vi "_CSMObj-Obtain CSM.vi"(7 "Allowed Messages (Empty For All)":string[](array[string]), 8 "error in (no error)":errorcluster, 11 "Requested Name":string) -> (0 "error out":errorcluster, 3 "CSMQ Out":T1)   [LabVIEW 2017, in "Communicable State Machine.lvlib"]
uses:
  Communicable State Machine.lvlib
  _CSMObj.ctl
  _CSMObj-Info.ctl
  Typedef/_CSM_MODE.ctl
  _CSMObj-Refs.ctl
  _CSMObj-Data.ctl
  Typedef/_CSM_MSG_TYPE.ctl
  Priority Queue/Priority Queue.ctl
  Typedef/_Cross CSM State Data.ctl
  Typedef/_Cross CSM State Response.ctl
  Typedef/_CSM_Response Source Message.ctl
  Priority Queue/def-Data(LowPRI-Q).ctl
  _CSMObj-ModeData.ctl
  Typedef/_CSM Status Change Event Data.ctl
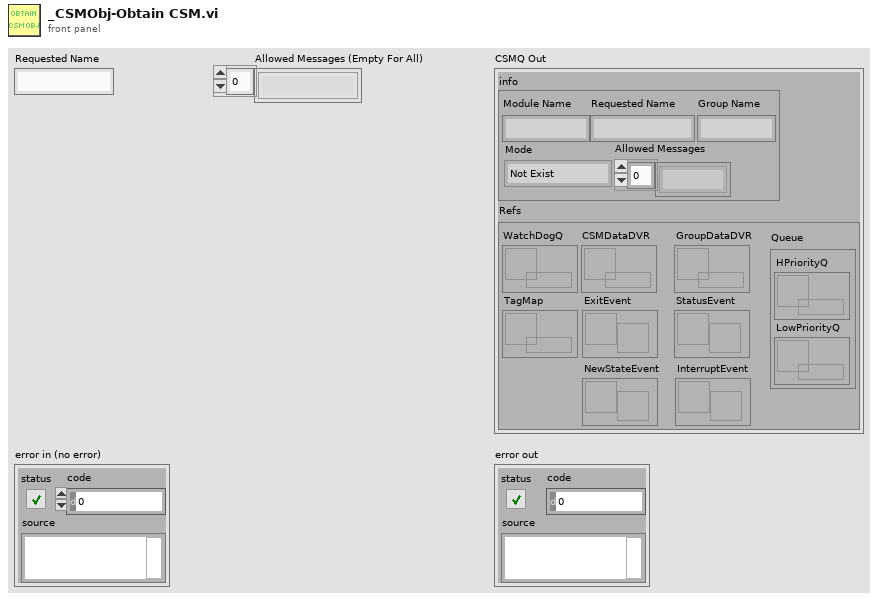
[diagram p1: front panel]
types:
  T1 = typedef "Communicable State Machine.lvlib/_CSMObj.ctl" = cluster{"info":T2, "Refs":T4}
  T2 = typedef "Communicable State Machine.lvlib/_CSMObj-Info.ctl" = cluster{"Module Name":string, "Requested Name":string, "Group Name":string, "Mode":T3, "Allowed Messages":string[]}
  T3 = typedef "Communicable State Machine.lvlib/_CSM_MODE.ctl" = enum16{"Not Exist", "Stand Alone", "CSM", "Worker", "Worker Agent", "Chain Node", "Chain"}
  T4 = typedef "Communicable State Machine.lvlib/_CSMObj-Refs.ctl" = cluster{"WatchDogQ":refnum<queue>, "CSMDataDVR":refnum<data-value>, "Queue":T5, "GroupDataDVR":refnum<data-value>, "TagMap":refnum<data-value>, "ExitEvent":refnum<user-event>, "NewStateEvent":refnum<user-event>, "StatusEvent":refnum<user-event>, "InterruptEvent":refnum<user-event>}
  T5 = typedef "Communicable State Machine.lvlib/Priority Queue.ctl" = cluster{"HPriorityQ":refnum<queue>, "LowPriorityQ":refnum<queue>}
  T6 = typedef "Communicable State Machine.lvlib/_CSMObj-Data.ctl" = cluster{"RemoteMessge?":bool, "error":errorcluster, "Return State":string, "Initialized":enum16{"Initializing", "Ready", "Exiting"}, "InternalRegistryRules":string[], "Return Msg Type":T7}
  T7 = typedef "Communicable State Machine.lvlib/_CSM_MSG_TYPE.ctl" = enum16{"Sync Message(-@)", "Async Message(->)", "Async without Response(->|)", "Async Response", "Broadcast(-><all>)", "Broadcast(-><status>)", "Broadcast(-><interrupt>)", "Append to JKISM States", "Append to JKISM States(High Priority)", "Broadcast(-><state>)", "<None>"}
  T8 = typedef "Communicable State Machine.lvlib/_CSMObj-ModeData.ctl" = cluster{"CSMDataDVR":refnum<data-value>[], "PriorityQueues":T5[], "Messages of Chain Nodes":cluster{"Module Name":string, "Allowed Messages":string[]}[], "Chain Message Mapping Map":variant, "SharedRegistryRules":string[]}
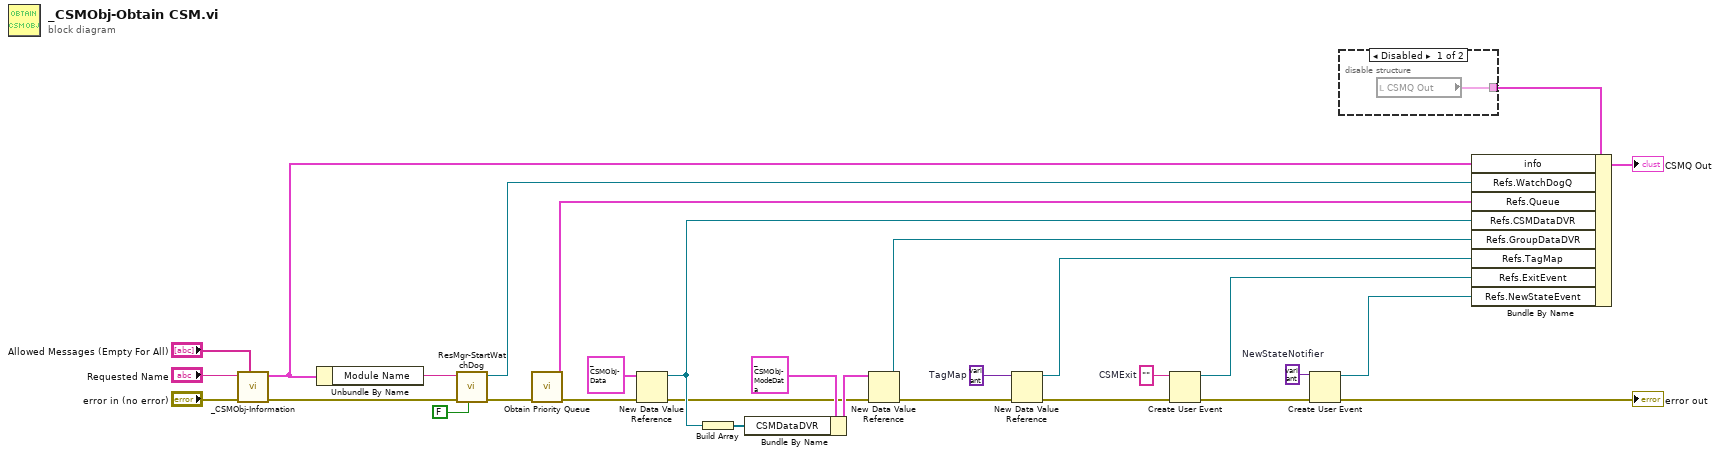
[diagram p0: block diagram]
diagram:
  w18 = variant  # NewStateNotifier
  w25 = variant  # TagMap
  w26 = ""  # CSMExit
  n1 = call "_CSMObj-Information.vi"("Allowed Messages (Empty For All)"="Allowed Messages (Empty For All)", "Error In"="error in (no error)", "Requested Name"="Requested Name") -> ("error out"=w4:errorcluster, "CSMO-Info"=w15:T2)  [unwired: 7 in]
  n2 = Unbundle By Name(w15) -> ("Module Name"=w19:string)
  n3 = call "ResMgr-StartWatchDog.vi"("Force?"=FALSE, "error in (no error)"=w4, "ModuleName"=w19) -> ("error out"=w5:errorcluster, "WatchDogQ"=w2:refnum<queue>)  [unwired: 7 in]
  n4 = call "Obtain Priority Queue.vi"("error in (no error)"=w5) -> ("error out"=w12:errorcluster, "Priority Queue"=w14:T5)  [unwired: 8 in, 1 out]
  n5 = New Data Value Reference(data value=T6 {"RemoteMessge?"=FALSE, "error"={"status"=FALSE, "code"=0, "source"=""}, "Return State"="", "Initialized"=enum."Initializing", "InternalRegistryRules"=[], "Return Msg Type"=enum."Sync Message(-@)"} ("CSMObj-Data"), error in=w12) -> (data value reference=w13:refnum<data-value>, error out=w11:errorcluster)
  n6 = Build Array(w13) -> (w20:refnum<data-value>[])
  n7 = Bundle By Name(cluster=T8 {"CSMDataDVR"=[], "PriorityQueues"=[], "Messages of Chain Nodes"=[], "Chain Message Mapping Map"=variant, "SharedRegistryRules"=[]} ("CSMObj-Data"), "CSMDataDVR"=w20) -> (w21:T8)
  n8 = New Data Value Reference(data value=w21, error in=w11) -> (data value reference=w10:refnum<data-value>, error out=w9:errorcluster)
  n9 = New Data Value Reference(data value=w25, error in=w9) -> (data value reference=w23:refnum<data-value>, error out=w7:errorcluster)
  n10 = Create User Event(user event datatype=w26, error in=w7) -> (user event=w24:refnum<user-event>, error out=w6:errorcluster)
  n11 = Create User Event(user event datatype=w18, error in=w6) -> (user event=w8:refnum<user-event>, error out=→"error out":errorcluster)
  n12 = disable-structure shown="Disabled" {
    disable-tunnel: [w31 _] -> w16
    frame Disabled {
      n13 = local read "CSMQ Out"() -> (w31:T1)
    }
    frame Enabled {
    }
  }
  n14 = Bundle By Name(cluster=w16, "info"=w15, "Refs.WatchDogQ"=w2, "Refs.Queue"=w14, "Refs.CSMDataDVR"=w13, "Refs.GroupDataDVR"=w10, "Refs.TagMap"=w23, "Refs.ExitEvent"=w24, "Refs.NewStateEvent"=w8) -> (→"CSMQ Out":T1)
